vi "Path as UTF-8 Path.vi"   [LabVIEW 2020, in "G-Unicode.lvlib"]
uses:
  G-Unicode.lvlib
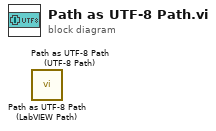
[diagram p0: block diagram]
diagram:
  n1 = call "Path as UTF-8 Path (LabVIEW Path).vi"() -> ()  [unwired: 10 in, 2 out]
  n2 = call "Path as UTF-8 Path (UTF-8 Path).vi"() -> ()  [unwired: 10 in, 2 out]
